vi "getDetections.vi"(0 "dl in":refnum<class "dl.lvclass">, 5 "numberofDetections":i32, 11 "error in (no error)":errorcluster) -> (4 "dl out":refnum<class "dl.lvclass">, 6 "return type":i32, 8 "detec":T1[](array[typedef]), 15 "error out":errorcluster)   [LabVIEW 2025, in "dl.lvlib" / "dl.lvclass"]
uses:
  dl.lvclass
  detect.ctl
  dl.lvclass/dl.ctl
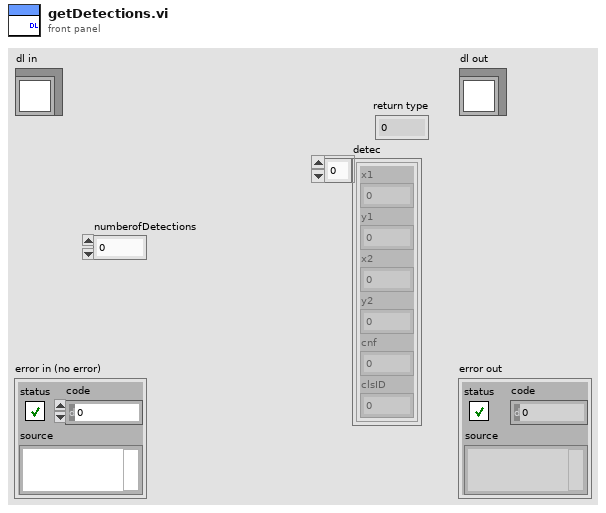
[diagram p1: front panel]
types:
  T1 = typedef "dl.lvlib/dl.lvclass/detect.ctl" = cluster{"x1":sgl, "y1":sgl, "x2":sgl, "y2":sgl, "cnf":sgl, "clsID":i32}
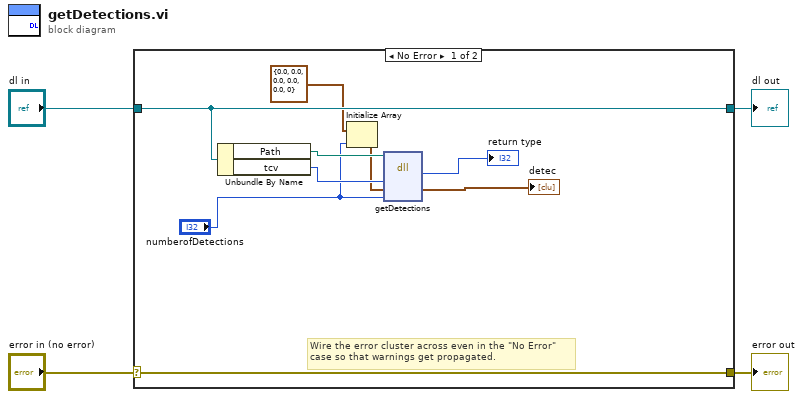
[diagram p0: block diagram]
diagram:
  n1 = case shown="No Error" "error in (no error)" {
    selector: "error in (no error)" -> [w13 w15]
    tunnel: [w13 w15] -> w3
    tunnel: [w12 w14] -> w1
    tunnel: "dl in" -> [w12 w14]
    frame No Error {
      # "Wire the error cluster across even in the \"No Error\"\ncase so that warnings get propagated."
      n2 = Unbundle By Name(w12) -> ("Path"=w11:path, "tcv"=w10:u64)
      n3 = Initialize Array(T1 {"x1"=0.0, "y1"=0.0, "x2"=0.0, "y2"=0.0, "cnf"=0.0, "clsID"=0}, "numberofDetections") -> (w6:T1[])
      n4 = dll-call lib="D:/Test/adslvPackageDev/Resources/TCV_Lib.dll" fn="getDetections"(path in=w11, "tcv"=w10, "detec"=w6, "numberofDetections"="numberofDetections") -> ("return type"=→"return type":i32, "detec"=→"detec":T1[])  [unwired: 4 in, 2 out]
    }
    frame Error {
    }
  }
  "error out" <- w3
  "dl out" <- w1
